vi "FPGA SPI_Globals.vi"() -> ()   [LabVIEW 2014]
uses:
  Controls/FPGA SPI_FPGA SPI State.ctl
  Controls/DacState.ctl
panel:
  in  "DacStateCmdByHost":T1
  in  "DacState":T1
  in  "setDACRegister":u32=1572792 caption="actRegister" format="%024b"
  in  "actDACRegister":u32=1572792 caption="actRegister" format="%024b"
  out "timeoutVoltSetDAC":bool
  in  "DAC Register 0V":u32=1572792 format="%024b"
  in  "SPI_Cmd":T2=enum."Configure"
  in  "SPI_Clock Divider":u32=20
  in  "SPI_CS Active State":bool caption="SPI_CS \nActive State"
  in  "SPI_CPOL":bool
  in  "SPI_CPHA":bool
  in  "SPI_CS":u8=128 format="%08b"
  in  "SPI_Total Bits":u16=8
  in  "SPI_Total Bytes":u16=1
  out "SPI_Done":bool
  out "SPI_Start":bool
  in  "SPI_Port":i8
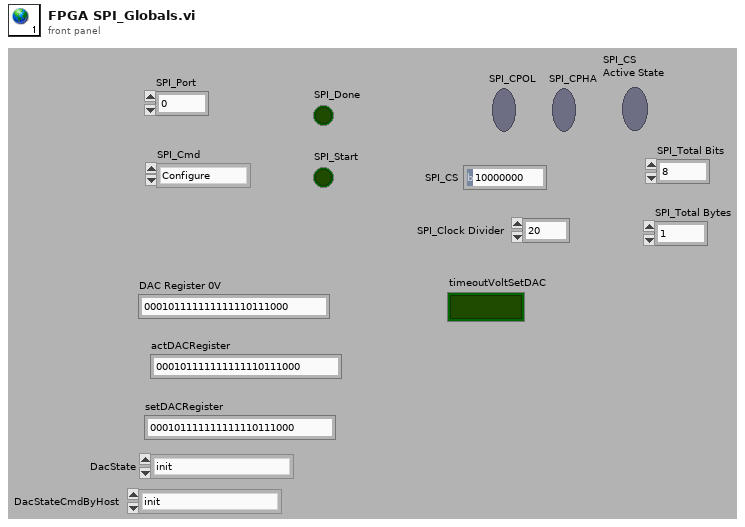
[diagram p1: front panel]
types:
  T1 = typedef "DacState.ctl" = enum16{"init", "idle", "setVolt", "error"}
  T2 = typedef "FPGA SPI_FPGA SPI State.ctl" = enum8{"Idle", "Read/Write SPI", "Configure"}
diagram:
